vi "JSON to Control Experiment Class.vi"(8 "error in (no error)":errorcluster, 10 "JSON":string, 11 "Control Experiment in":refnum<class "Control Experiment.lvclass">) -> (0 "error out":errorcluster, 1 "Unresolved on load":string[](array[string]), 2 "Loaded?":bool, 3 "Control Experiment out":refnum<class "Control Experiment.lvclass">)   [LabVIEW 2019, in "Control Experiment.lvclass"]
uses:
  Control Experiment.lvclass
  Typedefs/Control Experiment FGV.JSON--cluster.ctl
  Typedefs/Experiment Description--cluster.ctl
  Typedefs/Instruments--cluster.ctl
  Typedefs/Instrument Types--enum.ctl
  Typedefs/Wiring Description--cluster.ctl
  Control Experiment.lvclass/Control Experiment.ctl
  <userlib>/LevyLab/Instrument Framework/Instrument/Instrument.lvclass
  C:/Program Files/National Instruments/LabVIEW 2019/vi.lib/JKI/JKI SMO/SMO/SMO.lvclass
  <userlib>/LevyLab/Instrument Framework/Instrument/Instrument.lvclass/Instrument.ctl
  4736f241-b1b3-4803-b7c5-0c61b63bf0cc.vi
  <vilib>/JDP Science/JSONtext/JSON text to Variant.vi
  <vilib>/JDP Science/JSONtext/LVClass Serializer/JSONtext LVClass Serializer.lvclass
  Attributes/Instrument Attributes.lvlib
  <vilib>/JKI/JKI SMO/URI Parsing/URI.lvlib
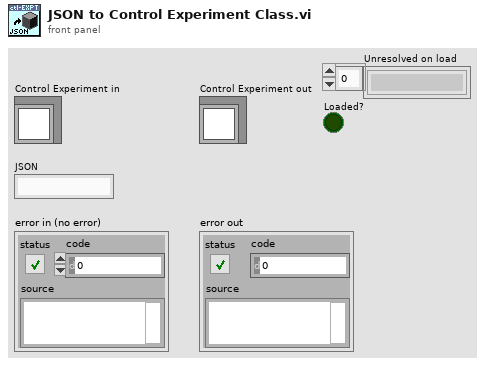
[diagram p1: front panel]
types:
  T1 = typedef "Control Experiment.lvclass/Control Experiment FGV.JSON--cluster.ctl" = cluster{"json":string, "Experiment":T2, "Wiring Configuration":T5}
  T2 = typedef "Control Experiment.lvclass/Experiment Description--cluster.ctl" = cluster{"User":string, "Device":string, "Device Path":path, "Device Description":string, "Experiment Path":path, "Experiment Description":string, "Instrument":string, "Instruments":T3[], "Sweep":cluster{"key":string, "value":variant}[]}
  T3 = typedef "Control Experiment.lvclass/Instruments--cluster.ctl" = cluster{"class path":path, "Address":string, "Type":T4}
  T4 = typedef "Control Experiment.lvclass/Instrument Types--enum.ctl" = enum16{"DAQ", "Amplifier", "Temperature", "Magnet", "Rotator", "Level", "Capacitance", "Delay Line", "Strain Cell", "VNA", "Source"}
  T5 = typedef "Control Experiment.lvclass/Wiring Description--cluster.ctl" = cluster{"Lockin Ch":i32[], "KH":cluster{"Electrodes":string[], "Labels":string[]}, "not KH":cluster{"Electrodes":string[], "Labels":string[]}}
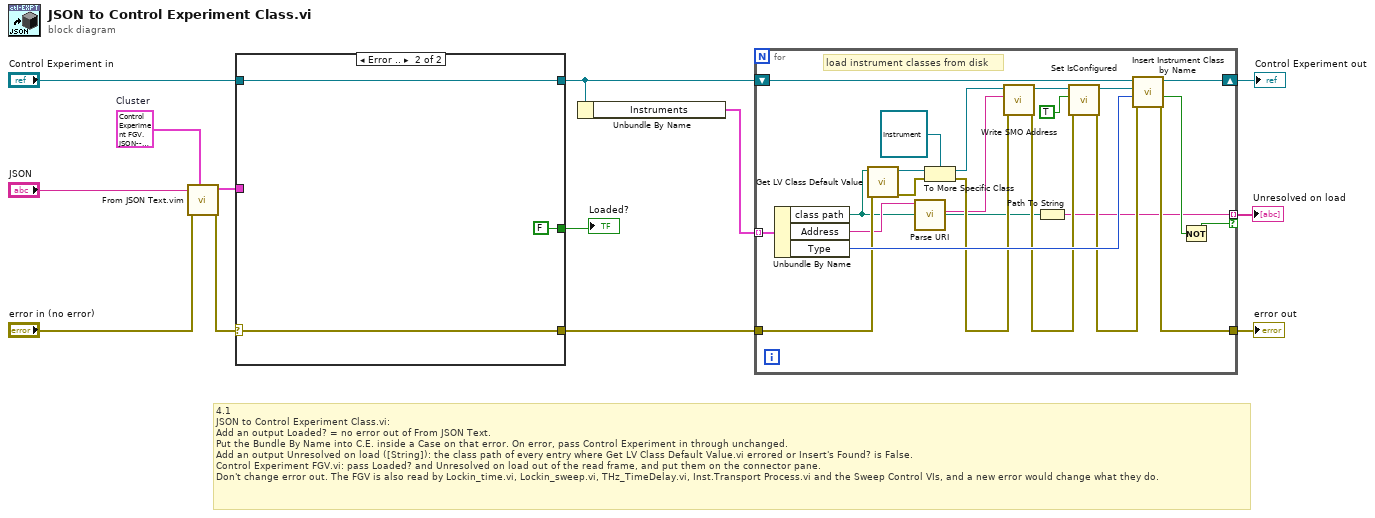
[diagram p0: block diagram]
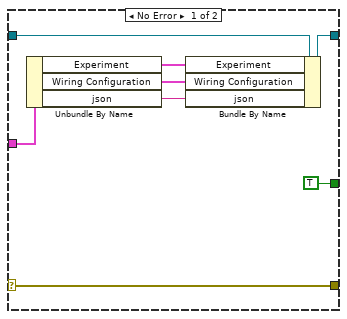
[diagram p2: hidden frame]
diagram:
  w7 = T1 {"json"="", "Experiment"={"User"="", "Device"="", "Device Path"=path "", "Device Description"="", "Experiment Path"=path "", "Experiment Description"="", "Instrument"="", "Instruments"=[], "Sweep"=[]}, "Wiring Configuration"={"Lockin Ch"=[], "KH"={"Electrodes"=[], "Labels"=[]}, "not KH"={"Electrodes"=[], "Labels"=[]}}}  # Cluster
  # "4.1\nJSON to Control Experiment Class.vi:\nAdd an output Loaded? = no error out of From JSON Text.\nPut the Bundle By Name into C.E. inside a Case on that error. On error, pass Control Experiment in through unchanged.\nAdd an output Unresolved on load ([String]): the class path of every entry where Get LV Class Default Value.vi errored or Insert's Found? is False.\nControl Experiment FGV.vi: pass Loaded? and Unresolved on load out of the read frame, and put them on the connector pane.\nDon't change error out. The FGV is also read by Lockin_time.vi, Lockin_sweep.vi, THz_TimeDelay.vi, Inst.Transport Process.vi and the Sweep Control VIs, and a new error would change what they do."
  n1 = call "From JSON Text.vim"("Data Type and Default Value"=w7, "error in (no error)"="error in (no error)", "JSON"="JSON") -> ("error out"=w3:errorcluster, "Data out"=w8:T1)  [unwired: 7 in]
  n2 = case shown="Error .." w3 {
    selector: w3 -> [w15 w24]
    tunnel: "Control Experiment in" -> [w21 w23]
    tunnel: w8 -> [w20 _]
    tunnel: [w16 w23] -> w5
    tunnel: [w15 w24] -> w4
    tunnel: [TRUE ("Loaded?") FALSE ("Loaded?")] -> w1
    frame No Error {
      n3 = Unbundle By Name(w20) -> ("Experiment"=w19:T2, "Wiring Configuration"=w18:T5, "json"=w17:string)
      n4 = Bundle By Name(cluster=w21, "Experiment"=w19, "Wiring Configuration"=w18, "json"=w17) -> (w16:refnum<class "Control Experiment.lvclass">)
    }
    frame Error {
    }
  }
  "Loaded?" <- w1
  n5 = Unbundle By Name(w5) -> ("Instruments"=w6:T3[])
  n6 = for {
    tunnel: w6 -> [w46] mode=indexing
    tunnel: w4 -> [w38]
    tunnel: [w40] -> w12
    shift-right: [w41] -> w9
    shift-left: w5 -> [w42]
    tunnel: [w26] -> w2 mode=indexing if=w25
    # "load instrument classes from disk"
    n7 = Unbundle By Name(w46) -> ("class path"=w28:path, "Address"=w30:string, "Type"=w39:T4)
    n8 = call <vilib>:"Get LV Class Default Value.vi"("error in (no error)"=w38, "class path"=w28) -> ("error out"=w43:errorcluster, "object"=w45:refnum<class>)  [unwired: 8 in]
    n9 = call <vilib>:"Parse URI.vi"("URI"=w30) -> ("address"=w29:string)  [unwired: 6 in, 4 out]
    n10 = To More Specific Class(target class=refnum<class "Instrument.lvclass"> refnum ("Instrument in"), reference=w45, error in=w43) -> (specific class reference=w36:refnum<class "Instrument.lvclass">, error out=w37:errorcluster)
    n11 = call <userlib>:"Write SMO Address.vi"("error in (no error)"=w37, "Address"=w29, "Instrument in"=w36) -> ("error out"=w33:errorcluster, "Instrument out"=w35:refnum<class "Instrument.lvclass">)  [unwired: 7 in]
    n12 = Path To String(path=w28) -> (string=w26:string)
    n13 = call "Set IsConfigured.vi"("error in (no error)"=w33, "IsConfigured?"=TRUE, "SMO"=w35) -> ("error out"=w32:errorcluster, "SMO out"=w34:refnum<class "Instrument.lvclass">)  [unwired: 7 in]
    n14 = call "Insert Instrument Class by Name.vi"("error in (no error)"=w32, "Type"=w39, "Instrument in"=w34, "Control Experiment in"=w42) -> ("error out"=w40:errorcluster, "Found?"=w27:bool, "Control Experiment out"=w41:refnum<class "Control Experiment.lvclass">)  [unwired: 4 in, 1 out]
    n15 = Not(x=w27) -> (.not. x?=w25:bool)
  }
  "Control Experiment out" <- w9
  "error out" <- w12
  "Unresolved on load" <- w2
